vi "FTW-File-Regex-Modify.vi"(0 "Filepath":path, 5 "Value Replacements":T1(array[cluster]), 11 "error in":errorcluster) -> (4 "Filepath out":path, 6 "Number of Replacements":i32[](array[numeric]), 15 "error out":errorcluster)   [LabVIEW 2013]
panel:
  # "Inputs"
  # "Outputs"
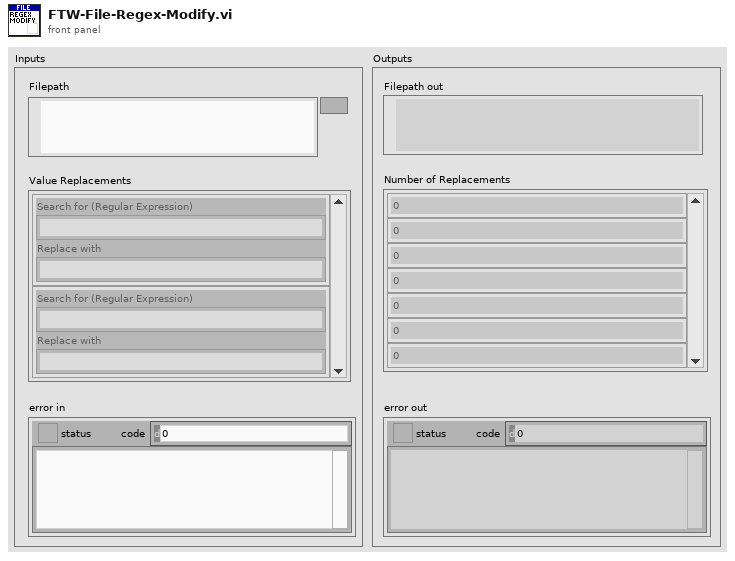
[diagram p1: front panel]
types:
  T1 = cluster{"Search for (Regular Expression)":string, "Replace with":string}[]
  T2 = enum16{"open", "replace", "create", "open or create", "replace or create", "replace or create with confirmation"}
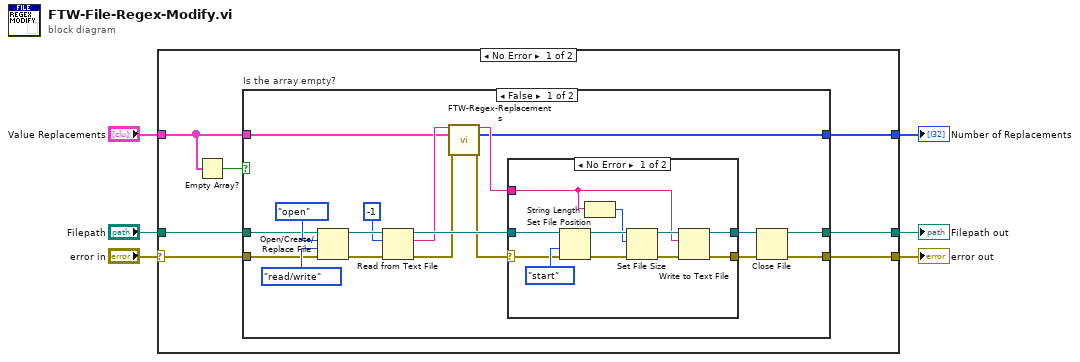
[diagram p0: block diagram]
diagram:
  n1 = case shown="No Error" "error in" {
    selector: "error in" -> [w12 w48]
    tunnel: [w13 w48] -> w6
    tunnel: "Filepath" -> [w11 w47]
    tunnel: "Value Replacements" -> [w8 _]
    tunnel: [w10 _] -> w2
    tunnel: [w9 w47] -> w1
    frame No Error {
      n2 = Empty Array?(array=w8) -> (empty?=w7:bool)
      n3 = case "Is the array empty?" shown="False" w7 {
        tunnel: [w23 w45] -> w13
        tunnel: w12 -> [w22 w45]
        tunnel: w11 -> [w21 w46]
        tunnel: w8 -> [w17 _]
        tunnel: [w16 _] -> w10
        tunnel: [w15 w46] -> w9
        frame False {
          n4 = Open/Create/Replace File(file path (use dialog)=w21, error in=w22, operation (0:open)=T2."open", access (0:read/write)=enum16{"read/write", "read-only", "write-only"}."read/write") -> (refnum out=w29:refnum<file>, error out=w28:errorcluster)  [unwired: 2 in, 1 out]
          n5 = Read from Text File(file (use dialog)=w29, count=-1, error in=w28) -> (refnum out=w26:refnum<file>, text=w20:string, error out=w18:errorcluster)  [unwired: 1 in, 1 out]
          n6 = call "FTW-Regex-Replacements.vi"("String"=w20, "Value Replacements"=w17, "error in"=w18) -> ("String out"=w19:string, "Number of Replacements"=w16:i32[], "error out"=w14:errorcluster)  [unwired: 10 in]
          n7 = case shown="No Error" w14 {
            selector: w14 -> [w38 w43]
            tunnel: w26 -> [w42 w44]
            tunnel: [w40 w44] -> w25
            tunnel: [w39 w43] -> w24
            tunnel: w19 -> [w33 _]
            frame No Error {
              n8 = Set File Position(refnum=w42, from (0:start)=enum16{"start", "end", "current"}."start", error in=w38) -> (refnum out=w37:refnum<file>, error out=w36:errorcluster)  [unwired: 1 in]
              n9 = String Length(string=w33) -> (length=w32:i32)
              n10 = Set File Size(4:w36, 6:w32, 7:w37) -> (0:w35:errorcluster, 3:w34:refnum<file>)
              n11 = Write to Text File(file (use dialog)=w34, text=w33, error in=w35) -> (refnum out=w40:refnum<file>, error out=w39:errorcluster)  [unwired: 1 in, 1 out]
            }
            frame Error {
            }
          }
          n12 = Close File(refnum=w25, error in=w24) -> (path=w15:path, error out=w23:errorcluster)
        }
        frame True {
        }
      }
    }
    frame Error {
    }
  }
  "error out" <- w6
  "Filepath out" <- w1
  "Number of Replacements" <- w2
